vi "FindTextInArray.vi"(10 "all rows":string[][](array[string]), 11 "String":string) -> (3 "Boolean":bool)   [LabVIEW 2024]
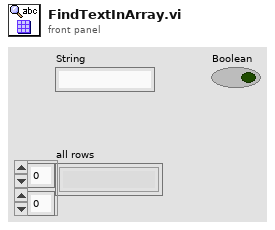
[diagram p1: front panel]
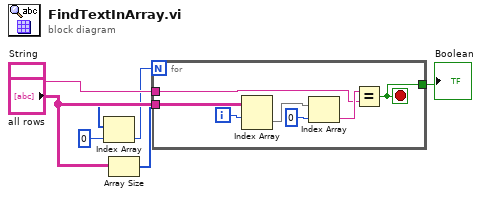
[diagram p0: block diagram]
diagram:
  n1 = Array Size(array="all rows") -> (size(s)=w2:i32[])
  n2 = Index Array(array=w2, index=0) -> (element=w4:i32)
  n3 = for {
    N: w4 -> [_]
    tunnel: "String" -> [w7]
    tunnel: "all rows" -> [w13]
    tunnel: [w8] -> w1
    i -> [w9]
    stop <- w8 stop-if-true
    n4 = Index Array(array=w13, index (row)=w9) -> (element=w10:string[])  [unwired: 1 in]
    n5 = Index Array(array=w10, index=0) -> (element=w12:string)
    n6 = Equal?(x=w12, y=w7) -> (x = y?=w8:bool)
  }
  "Boolean" <- w1
